vi "Permissions to U32.vi"(11 "permissions":T2) -> (3 "packed permissions":T1)   [LabVIEW 2013, in "Linux RT IPC.lvlib" / "Shared Memory.lvlib" / "Shared Memory.lvclass"]
doc: "Converts cluster of permissions to single packed U32 for C functions."
uses:
  Shared Memory.lvclass
  Controls/permissions group.ctl
  Controls/permissions.ctl
  Protected/Controls/C Types/mode_t.ctl
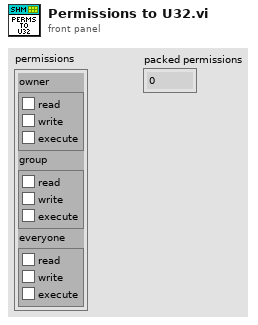
[diagram p1: front panel]
types:
  T1 = typedef "Linux RT IPC.lvlib/Shared Memory.lvlib/Shared Memory.lvclass/mode_t.ctl" = u32
  T2 = typedef "Linux RT IPC.lvlib/Shared Memory.lvlib/Shared Memory.lvclass/permissions group.ctl" = cluster{"owner":T3, "group":T3, "everyone":T3}
  T3 = typedef "Linux RT IPC.lvlib/Shared Memory.lvlib/Shared Memory.lvclass/permissions.ctl" = cluster{"read":bool, "write":bool, "execute":bool}
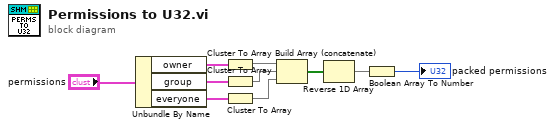
[diagram p0: block diagram]
diagram:
  n1 = Unbundle By Name("permissions") -> ("owner"=w3:T3, "group"=w4:T3, "everyone"=w5:T3)
  n2 = Cluster To Array(cluster=w3) -> (array=w6:bool[])
  n3 = Cluster To Array(cluster=w4) -> (array=w7:bool[])
  n4 = Cluster To Array(cluster=w5) -> (array=w8:bool[])
  n5 = Build Array (concatenate)(w6, w7, w8) -> (w9:bool[])
  n6 = Reverse 1D Array(array=w9) -> (reversed array=w10:bool[])
  n7 = Boolean Array To Number(Boolean array=w10) -> (number=→"packed permissions":u32)
